vi "Close.vi"(8 "error in":errorcluster, 11 "Alarming Strategy in":refnum<class "Alarming Actor Strategy.lvclass">) -> (0 "error out":errorcluster, 3 "Alarming Strategy out":refnum<class "Alarming Actor Strategy.lvclass">)   [LabVIEW 2024, in "Alarming Actor Strategy.lvclass"]
uses:
  Alarming Actor Strategy.lvclass
  Alarming Actor Strategy.lvclass/Alarming Actor Strategy.ctl
  <vilib>/ActorFramework/Message Enqueuer/Message Enqueuer.lvclass/Message Enqueuer.ctl
  <vilib>/ActorFramework/Stop Msg/Stop Msg.lvclass
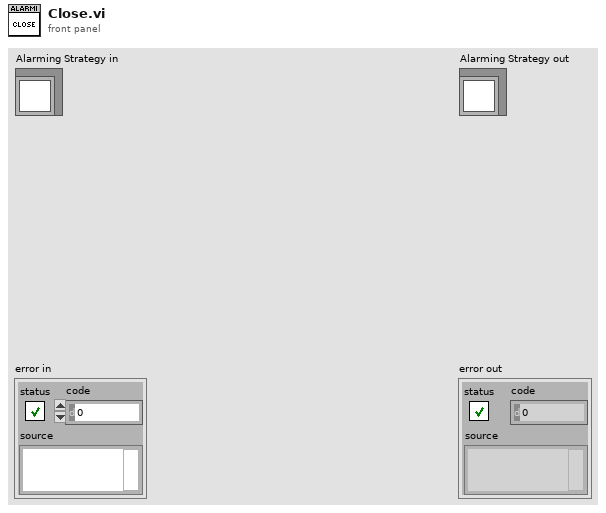
[diagram p1: front panel]
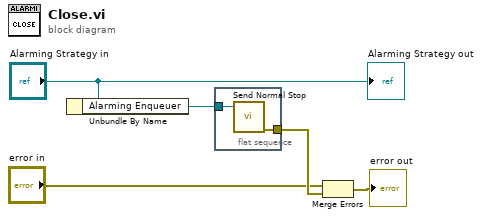
[diagram p0: block diagram]
diagram:
  n1 = Unbundle By Name("Alarming Strategy in") -> ("Alarming Enqueuer"=w4:refnum<class "Message Enqueuer.lvclass">)
  n2 = flat-sequence {
    tunnel: w4 -> [w7]
    tunnel: [w6] -> w3
    frame #0 {
      n3 = call <vilib>:"Send Normal Stop.vi"("Message Enqueuer"=w7) -> ("error out"=w6:errorcluster)  [unwired: 10 in]
    }
  }
  n4 = Merge Errors("error in", w3) -> (→"error out":errorcluster)
  "Alarming Strategy out" <- "Alarming Strategy in"
